vi "Autonomous Independent.vi"   [LabVIEW 2018]
doc: "This VI is called when autonomous begins, and will automatically be terminated when autonomous ends. You can carry out timed or sensor driven robot movement independently without needing to return to the caller."
uses:
  <vilib>/Rock Robotics/Network Tables/NT Read String.vi
  <vilib>/Rock Robotics/WPI/Utilities/WPI_GetSetVariantRefNum.vi
  <vilib>/Rock Robotics/WPI/RobotDrive/WPI_RobotDriveMecanumDrive_Cartesian.vi
  <vilib>/Rock Robotics/Network Tables/NT Write Numeric Array.vi
  <vilib>/Rock Robotics/Network Tables/NT Write Boolean Array.vi
  Robot Global Data.vi
panel:
  # "Be sure to right-click and choose Data Operations>>Make Current Value default if you want to save the array values with the VI"
types:
  T1 = typedef "WPI_RobotDriveDevRef.ctl" = cluster{"DevStatus":errorcluster, "Motors[]":T2[], "Square Inputs":bool, "Max Output":dbl}
  T2 = typedef "WPI_MotorControlDeviceRef.ctl" = cluster{"DeviceStatus":errorcluster, "Type":T3, "PWM":cluster{"PWM Channel":T4, "DeadBand":T5}, "CAN":cluster{"Device Number":u8, "SetOutput VI Ref":variant, "GetOutput VI Ref":variant, "Enable VI Ref":variant, "Disable VI Ref":variant, "Data":variant}, "Invert":bool, "DIO PWM":cluster{"PWM \"Enable\" Channel":T4, "DIOChannel":T6, "PWM Rate":dbl}}
  T3 = typedef "WPI_MotorControlType.ctl" = enum16{"PWM", "CAN", "DIO PWM"}
  T4 = typedef "FPGA_DIOPWMChannel.ctl" = enum8{"PWM 0", "PWM 1", "PWM 2", "PWM 3", "PWM 4", "PWM 5", "PWM 6", "PWM 7", "PWM 8", "PWM 9", "PWM MXP 0", "PWM MXP 1", "PWM MXP 2", "PWM MXP 3", "PWM MXP 4", "PWM MXP 5", "PWM MXP 6", "PWM MXP 7", "PWM MXP 8", "PWM MXP 9", "Invalid"}
  T5 = typedef "WPI_PWMDeadband.ctl" = cluster{"Name":string, "maxPositivePwm":i32, "minPositivePwm":i32, "centerPwm":i32, "maxNegativePwm":i32, "minNegativePwm":i32, "angularRange":u16}
  T6 = typedef "FPGA_DIOChannel.ctl" = enum8{"DIO 0", "DIO 1", "DIO 2", "DIO 3", "DIO 4", "DIO 5", "DIO 6", "DIO 7", "DIO 8", "DIO 9", "DIO MXP 0", "DIO MXP 1", "DIO MXP 2", "DIO MXP 3", "DIO MXP 4", "DIO MXP 5", "DIO MXP 6", "DIO MXP 7", "DIO MXP 8", "DIO MXP 9", "DIO MXP 10", "DIO MXP 11", "DIO MXP 12", "DIO MXP 13", "DIO MXP 14", "DIO MXP 15", "SPI Port CS1", "SPI Port CS2", "SPI Port CS3", "SPI Port MISO", "SPI Port MOSI", "Invalid"}
  T7 = typedef "WPI_JoystickDevRef.ctl" = cluster{"Device":T8}
  T8 = typedef "WPI_JoystickDeviceEnum.ctl" = enum16{"USB 0", "USB 1", "USB 2", "USB 3", "USB 4", "USB 5"}
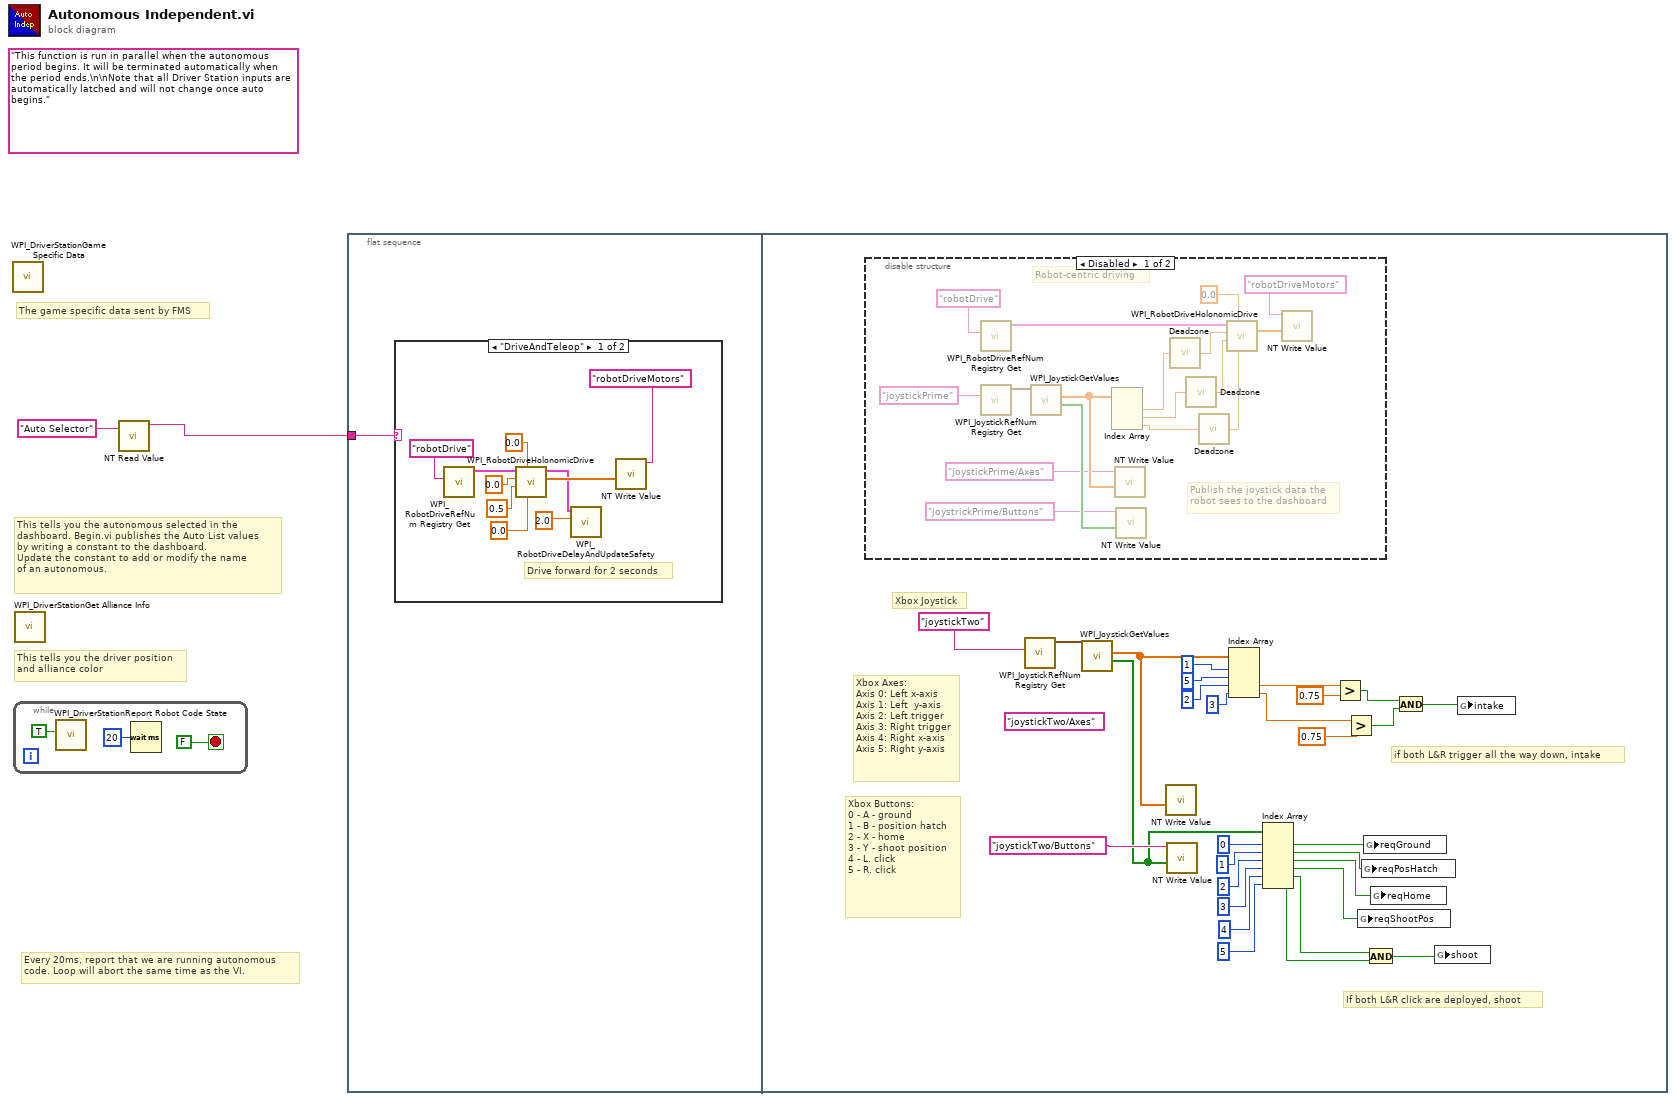
[diagram p0: block diagram]
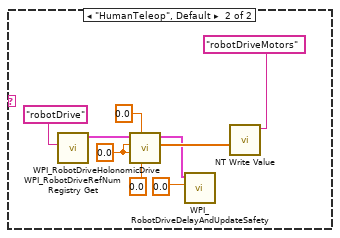
[diagram p2: hidden frame]
diagram:
  (unwired) "This function is run in parallel when the autonomous period begins. It will be terminated automatically when the period ends.\n\nNote that all Driver Station inputs are automatically latched and will not change once auto begins."
  # "The game specific data sent by FMS"
  # "This tells you the autonomous selected in the \ndashboard. Begin.vi publishes the Auto List values\nby writing a constant to the dashboard.\nUpdate the constant to add or modify the name\nof an autonomous."
  # "Every 20ms, report that we are running autonomous\ncode. Loop will abort the same time as the VI."
  # "This tells you the driver position\nand alliance color"
  n1 = call <vilib>:"WPI_DriverStationGame Specific Data.vi"() -> ()  [unwired: 11 in, 1 out]
  n2 = while {
    stop <- FALSE stop-if-true
    n3 = call <vilib>:"WPI_DriverStationReport Robot Code State.vi"("Autonomous"=TRUE) -> ()  [unwired: 10 in, 1 out]
    n4 = Wait (ms)(milliseconds to wait=u32 20) -> ()  [unwired: 1 out]
  }
  n5 = call <vilib>:"WPI_DriverStationGet Alliance Info.vi"() -> ()  [unwired: 12 out]
  n6 = call-poly <vilib>:"NT Read Value.vi"("Name"="Auto Selector") -> ("String"=w1:string)  [unwired: 9 in, 1 out]
  n7 = flat-sequence {
    tunnel: w1 -> [w6]
    frame #0 {
      n8 = case shown="\"DriveAndTeleop\"" w6 {
        frame "DriveAndTeleop" {
          # "Drive forward for 2 seconds"
          n9 = call <vilib>:"WPI_RobotDriveRefNum Registry Get.vi"("refnum name"="robotDrive") -> ("RobotDriveDevRef"=w15:T1)  [unwired: 1 in, 9 out]
          n10 = call-poly <vilib>:"WPI_RobotDriveHolonomicDrive.vi"("Rotation"=0.0, "Gyro Angle"=0.0, "Y"=0.5, "X"=0.0, "RobotDriveDevRef"=w15) -> ("Motor Values"=w12:dbl[], "RobotDriveDevRef"=w11:T1)  [unwired: 4 in, 1 out]
          n11 = call <vilib>:"WPI_RobotDriveDelayAndUpdateSafety.vi"("Delay (s)"=2.0, "RobotDriveDevRef"=w11) -> ()  [unwired: 8 in, 2 out]
          n12 = call-poly <vilib>:"NT Write Value.vi"("Numeric Array"=w12, "Name"="robotDriveMotors") -> ()  [unwired: 9 in, 1 out]
        }
        frame "HumanTeleop", Default {
          w18 = 0.0 ("Y")
          n13 = call <vilib>:"WPI_RobotDriveRefNum Registry Get.vi"("refnum name"="robotDrive") -> ("RobotDriveDevRef"=w24:T1)  [unwired: 1 in, 9 out]
          n14 = call-poly <vilib>:"WPI_RobotDriveHolonomicDrive.vi"("Rotation"=0.0, "Gyro Angle"=0.0, "Y"=w18, "X"=w18, "RobotDriveDevRef"=w24) -> ("Motor Values"=w22:dbl[], "RobotDriveDevRef"=w21:T1)  [unwired: 4 in, 1 out]
          n15 = call <vilib>:"WPI_RobotDriveDelayAndUpdateSafety.vi"("Delay (s)"=0.0, "RobotDriveDevRef"=w21) -> ()  [unwired: 8 in, 2 out]
          n16 = call-poly <vilib>:"NT Write Value.vi"("Numeric Array"=w22, "Name"="robotDriveMotors") -> ()  [unwired: 9 in, 1 out]
        }
      }
    }
    frame #1 {
      (unwired) "joystickTwo/Axes" ("Name")
      # "if both L&R trigger all the way down, intake"
      # "If both L&R click are deployed, shoot"
      # "Xbox Buttons:\n0 - A - ground\n1 - B - position hatch\n2 - X - home\n3 - Y - shoot position\n4 - L. click\n5 - R. click"
      # "Xbox Joystick"
      # "Xbox Axes:\nAxis 0: Left x-axis\nAxis 1: Left  y-axis\nAxis 2: Left trigger\nAxis 3: Right trigger\nAxis 4: Right x-axis\nAxis 5: Right y-axis"
      n17 = disable-structure shown="Disabled" {
        frame Disabled {
          # "Publish the joystick data the\nrobot sees to the dashboard"
          # "Robot-centric driving"
          n18 = call <vilib>:"WPI_RobotDriveRefNum Registry Get.vi"("refnum name"="robotDrive") -> ("RobotDriveDevRef"=w67:T1)  [unwired: 1 in, 9 out]
          n19 = call <vilib>:"WPI_JoystickRefNum Registry Get.vi"("refnum name"="joystickPrime") -> ("JoystickDevRef"=w68:T7)  [unwired: 1 in, 9 out]
          n20 = call <vilib>:"WPI_JoystickGetValues.vi"("JoystickDevRef"=w68) -> ("Buttons"=w70:bool[], "Axes"=w69:dbl[])  [unwired: 6 in, 3 out]
          n21 = Index Array(array=w69) -> (element #1=w59:dbl, element #2=w57:dbl, element #3=w56:dbl)  [unwired: 3 in]
          n22 = call-poly <vilib>:"NT Write Value.vi"("Numeric Array"=w69, "Name"="joystickPrime/Axes") -> ()  [unwired: 9 in, 1 out]
          n23 = call-poly <vilib>:"NT Write Value.vi"("Boolean Array"=w70, "Name"="joystrickPrime/Buttons") -> ()  [unwired: 9 in, 1 out]
          n24 = call "Deadzone.vi"("valInput"=w59) -> ("valOutput"=w60:dbl)
          n25 = call "Deadzone.vi"("valInput"=w57) -> ("valOutput"=w58:dbl)
          n26 = call "Deadzone.vi"("valInput"=w56) -> ("valOutput"=w55:dbl)
          n27 = call-poly <vilib>:"WPI_RobotDriveHolonomicDrive.vi"("Rotation"=w55, "Gyro Angle"=0.0, "Y"=w58, "X"=w60, "RobotDriveDevRef"=w67) -> ("Motor Values"=w71:dbl[])  [unwired: 4 in, 2 out]
          n28 = call-poly <vilib>:"NT Write Value.vi"("Numeric Array"=w71, "Name"="robotDriveMotors") -> ()  [unwired: 9 in, 1 out]
        }
        frame Enabled {
        }
      }
      n29 = call <vilib>:"WPI_JoystickRefNum Registry Get.vi"("refnum name"="joystickTwo") -> ("JoystickDevRef"=w52:T7)  [unwired: 1 in, 9 out]
      n30 = call <vilib>:"WPI_JoystickGetValues.vi"("JoystickDevRef"=w52) -> ("Buttons"=w48:bool[], "Axes"=w51:dbl[])  [unwired: 6 in, 3 out]
      n31 = call-poly <vilib>:"NT Write Value.vi"("Numeric Array"=w51) -> ()  [unwired: 10 in, 1 out]
      n32 = call-poly <vilib>:"NT Write Value.vi"("Boolean Array"=w48, "Name"="joystickTwo/Buttons") -> ()  [unwired: 9 in, 1 out]
      n33 = Index Array(array=w51, index #1=1 ("index"), index #2=5 ("index"), index #3=2 ("index"), index #4=3 ("index")) -> (element #3=w32:dbl, element #4=w29:dbl)  [unwired: 2 out]
      n34 = Index Array(array=w48, index #1=0 ("index"), index #2=1 ("index"), index #3=2 ("index"), index #4=3 ("index"), index #5=4 ("index"), index #6=5 ("index")) -> (element #1=w47:bool, element #2=w46:bool, element #3=w39:bool, element #4=w38:bool, element #5=w36:bool, element #6=w35:bool)
      n35 = Greater?(x=w32, y=0.75) -> (0:w28:bool)
      n36 = Greater?(x=w29, y=0.75) -> (0:w27:bool)
      n37 = global write "Robot Global Data.vi" "reqShootPos"(w38) -> ()
      n38 = global write "Robot Global Data.vi" "reqPosHatch"(w46) -> ()
      n39 = global write "Robot Global Data.vi" "reqGround"(w47) -> ()
      n40 = And(x=w36, y=w35) -> (x .and. y?=w37:bool)
      n41 = global write "Robot Global Data.vi" "reqHome"(w39) -> ()
      n42 = And(x=w28, y=w27) -> (x .and. y?=w26:bool)
      n43 = global write "Robot Global Data.vi" "shoot"(w37) -> ()
      n44 = global write "Robot Global Data.vi" "intake"(w26) -> ()
    }
  }
